vi "GetVision.vi"() -> (1 "Particle Measurements\n         X             Y           area":dbl[][](array[numeric]) format="%_3f")   [LabVIEW 2017]
panel:
  in  "Selection Values (Filter nonRound Particles)":T1(array[cluster])=[{"Measurement Parameter"=55, "Range Lower Value"=0.800000011920929, "Range Upper Value"=1.2000000476837158, "Range"=FALSE, "Measurement Type"=FALSE}] {"Measurement Parameter" items=["Center of Mass X", "Center of Mass Y", "First Pixel X", "First Pixel Y", "Bounding Rect Left", "Bounding Rect Top", "Bounding Rect Right", "Bounding Rect Bottom", "Max Feret Diameter Start X", "Max Feret Diameter Start Y", "Max Feret Diameter End X", "Max Feret Diameter End Y", "Max Horiz. Segment Length Left", "Max Horiz. Segment Length Right", "Max Horiz. Segment Length Row", "-", "Bounding Rect Width", "Bounding Rect Height", "Bounding Rect Diagonal", "Perimeter", "Convex Hull Perimeter", "Holes' Perimeter", "Max Feret Diameter", "Equivalent Ellipse Major Axis", "Equivalent Ellipse Minor Axis", "Equivalent Ellipse Minor Axis (Feret)", "Equivalent Rect Long Side", "Equivalent Rect Short Side", "Equivalent Rect Diagonal", "Equivalent Rect Short Side (Feret)", "Average Horiz. Segment Length", "Average Vert. Segment Length", "Hydraulic Radius", "Waddel Disk Diameter", "-", "Area", "Holes' Area", "Particle & Holes' Area", "Convex Hull Area", "Image Area", "-", "Number of Holes", "Number of Horiz. Segments", "Number of Vert. Segments", "-", "Orientation", "Max Feret Diameter Orientation", "-", "% Area/Image Area", "% Area/(Particle & Holes' Area)", "Ratio of Equivalent Ellipse Axes", "Ratio of Equivalent Rect Sides", "-", "Elongation Factor", "Compactness Factor", "Heywood Circularity Factor", "Type Factor", "-", "Sum X", "Sum Y", "Sum XX", "Sum XY", "Sum YY", "Sum XXX", "Sum XXY", "Sum XYY", "Sum YYY", "-", "Moment of Inertia XX", "Moment of Inertia XY", "Moment of Inertia YY", "Moment of Inertia XXX", "Moment of Inertia XXY", "Moment of Inertia XYY", "Moment of Inertia YYY", "Norm. Moment of Inertia XX", "Norm. Moment of Inertia XY", "Norm. Moment of Inertia YY", "Norm. Moment of Inertia XXX", "Norm. Moment of Inertia XXY", "Norm. Moment of Inertia XYY", "Norm. Moment of Inertia YYY", "Hu Moment 1", "Hu Moment 2", "Hu Moment 3", "Hu Moment 4", "Hu Moment 5", "Hu Moment 6", "Hu Moment 7"]}
  in  "Camera Brightness":i64=125 min=30 max=255 step=1
  out "Raw Image Out":T2(plugin-control)
  out "Processed Image Out":T2(plugin-control)
  # "Circularity Filter"
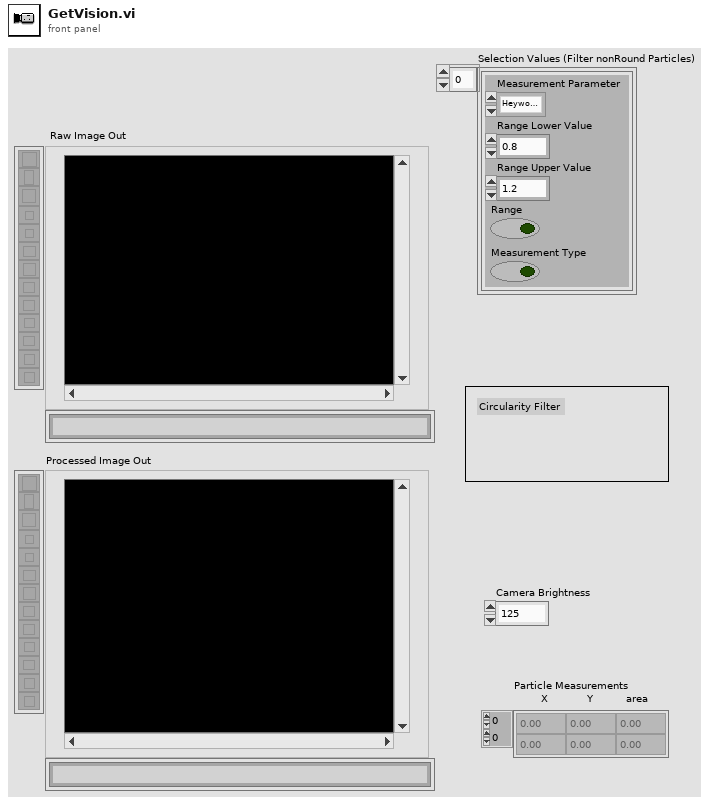
[diagram p1: front panel]
types:
  T1 = cluster{"Measurement Parameter":i32, "Range Lower Value":dbl, "Range Upper Value":dbl, "Range":bool, "Measurement Type":bool}[]
  T2 = typedef "IMAQ Image.ctl" = refnum<image>
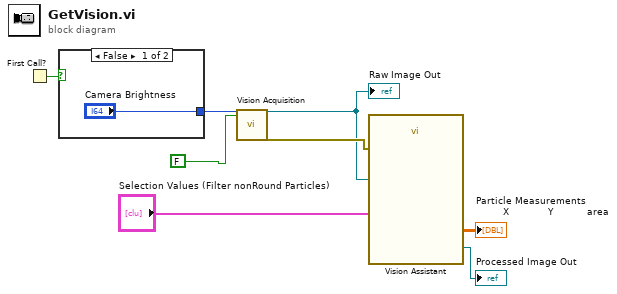
[diagram p0: block diagram]
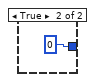
[diagram p2: hidden frame]
diagram:
  n1 = First Call?() -> (First Call?: T/F=w2:bool)
  n2 = case shown="False" w2 {
    tunnel: ["Camera Brightness" i64 0 ("Brightness::Value")] -> w4
    frame False {
    }
    frame True {
    }
  }
  n3 = call "Vision Acquisition"("Brightness::Value"=w4, "Log Image"=FALSE) -> ("Image Out"=w5:T2, "error out"=w7:errorcluster)  [unwired: 22 in, 2 out]
  "Raw Image Out" <- w5
  n4 = call "Vision Assistant"("Image In"=w5, "Selection Values (Filter nonRound Particles)"="Selection Values (Filter nonRound Particles)", "error in"=w7) -> ("Image Out"=→"Processed Image Out":T2, "Particle Measurements (Pixels) (Particle Analysis 1)"=→"Particle Measurements\n         X             Y           area":dbl[][])  [unwired: 22 in, 1 out]
